vi "Three-PWM.vi"(8 "Error In":errorcluster, 11 "Dutycycle(%)":dbl[](array[numeric])) -> (0 "Error Out":errorcluster)   [LabVIEW 2019]
uses:
  <vilib>/Utility/error.llb/Error Cluster From Error Code.vi
  <vilib>/myRIO/Common/Instrument Driver Framework/myRIO v1.0/DIO/vis/myRIO v1.0 Write DIO.vi
  <vilib>/myRIO/Common/Instrument Driver Framework/myRIO v1.0/PWM/vis/myRIO v1.0 Write PWM.vi
  <vilib>/myRIO/Instrument Drivers/Onboard IO/PWM/PWM.lvlib
  <vilib>/myRIO/Instrument Drivers/Onboard IO/DIO/DIO.lvlib
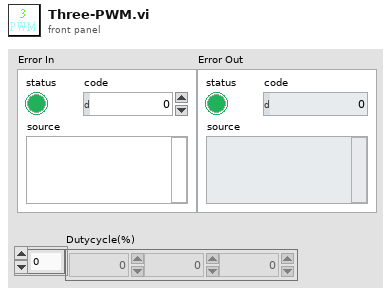
[diagram p1: front panel]
types:
  T1 = cluster{"馬達PWM腳位":tag, "馬達DIR腳位":tag[], "馬達Encoder角位":tag}[]
  T2 = cluster{"馬達PWM腳位":tag, "馬達DIR腳位":tag[], "馬達Encoder角位":tag}
  T3 = typedef "PWM.lvlib/PWM Reference.ctl" = cluster{"myRIO Reference":T4, "PWM Channels Enum":T8, "PWM Configuration":T9}
  T4 = typedef "myRIO Generic Hardware Reference.ctl" = cluster{"myRIO Model":T5, "myRIO Hardware Reference":T6}
  T5 = typedef "Hardware Version Enum.ctl" = enum16{"Unknown", "myRIO-1900", "myRIO-1950", "roboRIO", "NI ELVIS RIO CM", "ELVIS III"}
  T6 = typedef "myRIO v1.0 Reference.ctl" = cluster{"Generic FPGA Reference":T7, "Allow multiple opens":bool}
  T7 = typedef "Generic FPGA Reference.ctl" = refnum<k20>
  T8 = typedef "PWM Channels Enum.ctl" = enum16{"Not Connected", "C/PWM0", "C/PWM1", "A/PWM0", "A/PWM1", "A/PWM2", "A/PWM3", "A/PWM4", "A/PWM5", "A/PWM6", "A/PWM7", "A/PWM8", "A/PWM9", "A/PWM10", "A/PWM11", "A/PWM12", "A/PWM13", "A/PWM14", "A/PWM15", "A/PWM16", "A/PWM17", "A/PWM18", "A/PWM19", "B/PWM0", "B/PWM1", "B/PWM2", "B/PWM3", "B/PWM4", "B/PWM5", "B/PWM6", "B/PWM7", "B/PWM8", "B/PWM9", "B/PWM10", "B/PWM11", "B/PWM12", "B/PWM13", "B/PWM14", "B/PWM15", "B/PWM16", "B/PWM17", "B/PWM18", "B/PWM19", "PWM/PWM0", "PWM/PWM1", "PWM/PWM2", "PWM/PWM3", "PWM/PWM4", "PWM/PWM5", "PWM/PWM6", "PWM/PWM7", "PWM/PWM8", "PWM/PWM9"}
  T9 = typedef "PWM.lvlib/PWM Configuration.ctl" = cluster{"Frequency":dbl, "Duty Cycle":dbl}
  T10 = typedef "DIO.lvlib/DIO Reference.ctl" = cluster{"myRIO Reference":T4, "DIO Channels List":T11}
  T11 = typedef "DIO Channels List.ctl" = T12[]
  T12 = typedef "DIO Channels Enum.ctl" = enum16{"Not Connected", "C/DIO0", "C/DIO1", "C/DIO2", "C/DIO3", "C/DIO4", "C/DIO5", "C/DIO6", "C/DIO7", "A/DIO0", "A/DIO1", "A/DIO2", "A/DIO3", "A/DIO4", "A/DIO5", "A/DIO6", "A/DIO7", "A/DIO8", "A/DIO9", "A/DIO10", "A/DIO11", "A/DIO12", "A/DIO13", "A/DIO14", "A/DIO15", "A/DIO16", "A/DIO17", "A/DIO18", "A/DIO19", "B/DIO0", "B/DIO1", "B/DIO2", "B/DIO3", "B/DIO4", "B/DIO5", "B/DIO6", "B/DIO7", "B/DIO8", "B/DIO9", "B/DIO10", "B/DIO11", "B/DIO12", "B/DIO13", "B/DIO14", "B/DIO15", "B/DIO16", "B/DIO17", "B/DIO18", "B/DIO19", "LED0", "LED1", "LED2", "LED3", "Button0", "DIO/DIO0", "DIO/DIO1", "DIO/DIO2", "DIO/DIO3", "DIO/DIO4", "DIO/DIO5", "DIO/DIO6", "DIO/DIO7", "DIO/DIO8", "DIO/DIO9", "SPI/CS0", "SPI/CS1", "SPI/CS2", "SPI/CS3", "LED RADIO (Green)", "LED RADIO (Red)", "LED COMM (Green)", "LED COMM (Red)", "LED MODE (Green)", "LED MODE (Red)"}
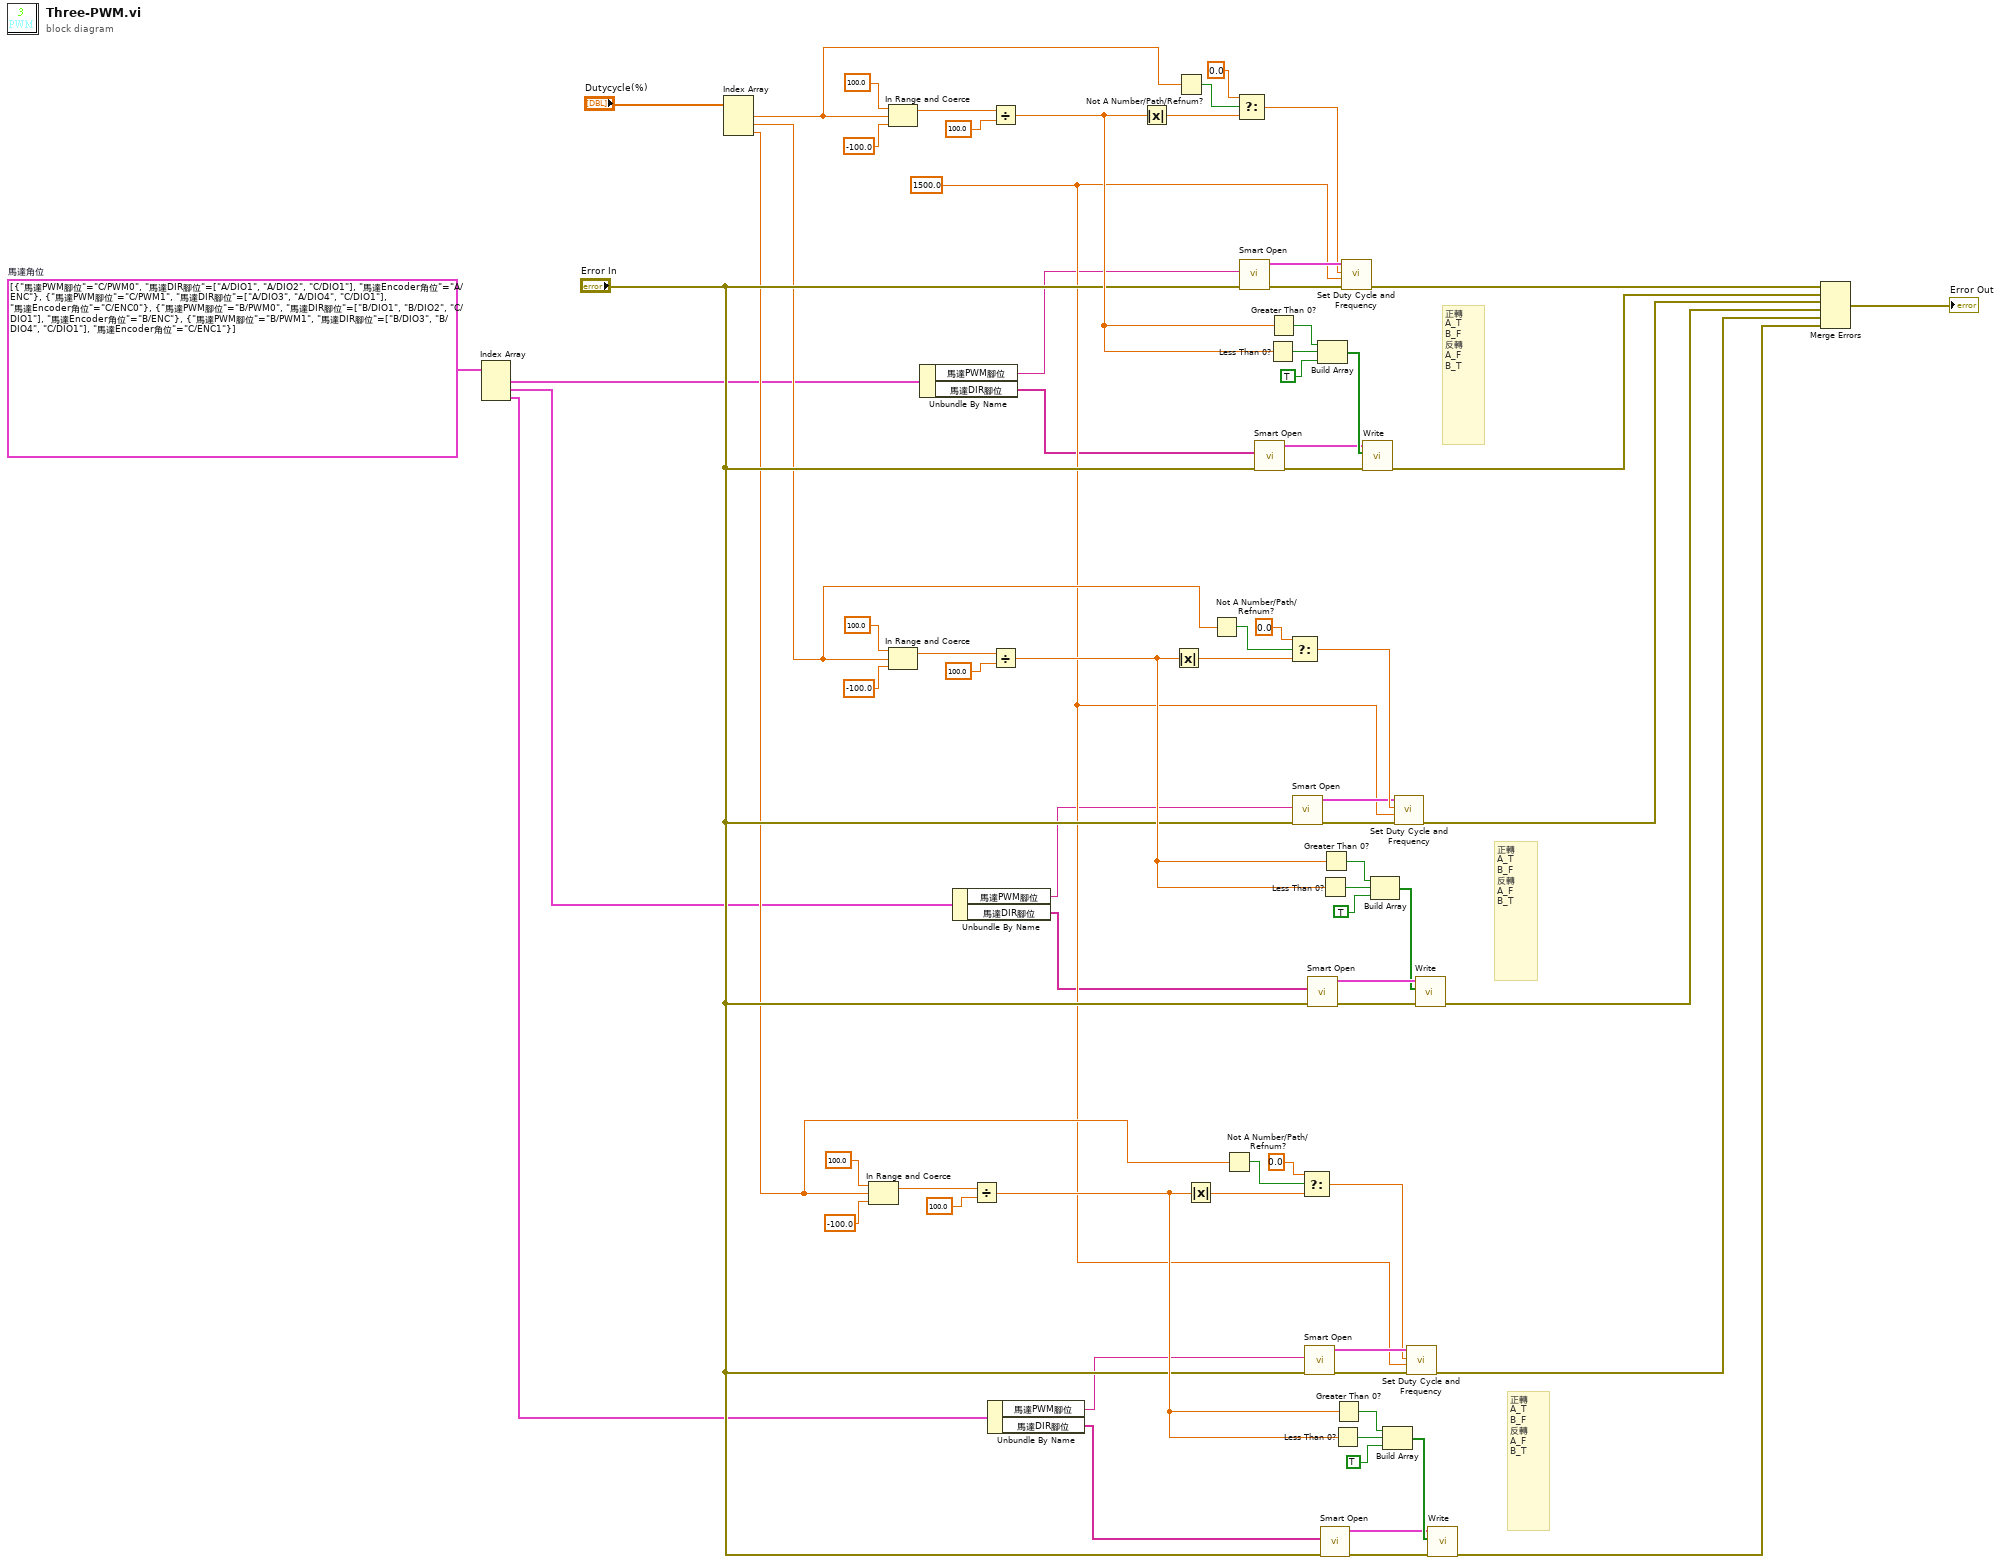
[diagram p0: block diagram]
diagram:
  w10 = T1 [{"馬達PWM腳位"="C/PWM0", "馬達DIR腳位"=["A/DIO1", "A/DIO2", "C/DIO1"], "馬達Encoder角位"="A/ENC"}, {"馬達PWM腳位"="C/PWM1", "馬達DIR腳位"=["A/DIO3", "A/DIO4", "C/DIO1"], "馬達Encoder角位"="C/ENC0"}, {"馬達PWM腳位"="B/PWM0", "馬達DIR腳位"=["B/DIO1", "B/DIO2", "C/DIO1"], "馬達Encoder角位"="B/ENC"}, {"馬達PWM腳位"="B/PWM1", "馬達DIR腳位"=["B/DIO3", "B/DIO4", "C/DIO1"], "馬達Encoder角位"="C/ENC1"}]  # 馬達角位
  w11 = 1500.0 ("Frequency [Hz]")
  # "正轉\nA_T\nB_F\n反轉\nA_F\nB_T"
  # "正轉\nA_T\nB_F\n反轉\nA_F\nB_T"
  # "正轉\nA_T\nB_F\n反轉\nA_F\nB_T"
  n1 = Index Array(array=w10) -> (element #1=w9:T2, element #2=w7:T2, element #3=w8:T2)  [unwired: 3 in]
  n2 = Index Array(array="Dutycycle(%)") -> (element #1=w14:dbl, element #2=w13:dbl, element #3=w12:dbl)  [unwired: 3 in]
  n3 = In Range and Coerce(upper limit=100.0, x=w12, lower limit=-100.0) -> (coerced(x)=w29:dbl)  [unwired: 1 out]
  n4 = In Range and Coerce(upper limit=100.0, x=w14, lower limit=-100.0) -> (coerced(x)=w63:dbl)  [unwired: 1 out]
  n5 = In Range and Coerce(upper limit=100.0, x=w13, lower limit=-100.0) -> (coerced(x)=w46:dbl)  [unwired: 1 out]
  n6 = Unbundle By Name(w9) -> ("馬達PWM腳位"=w5:tag, "馬達DIR腳位"=w6:tag[])
  n7 = Unbundle By Name(w7) -> ("馬達PWM腳位"=w3:tag, "馬達DIR腳位"=w4:tag[])
  n8 = Divide(x=w29, y=100.0) -> (x/y=w25:dbl)
  n9 = Unbundle By Name(w8) -> ("馬達PWM腳位"=w1:tag, "馬達DIR腳位"=w2:tag[])
  n10 = Divide(x=w63, y=100.0) -> (x/y=w59:dbl)
  n11 = Divide(x=w46, y=100.0) -> (x/y=w50:dbl)
  n12 = Absolute Value(x=w59) -> (abs(x)=w56:dbl)
  n13 = Absolute Value(x=w50) -> (abs(x)=w53:dbl)
  n14 = Not A Number/Path/Refnum?(number/path/refnum=w14) -> (NaN/Path/Refnum?=w58:bool)
  n15 = Absolute Value(x=w25) -> (abs(x)=w22:dbl)
  n16 = Not A Number/Path/Refnum?(number/path/refnum=w13) -> (NaN/Path/Refnum?=w51:bool)
  n17 = Not A Number/Path/Refnum?(number/path/refnum=w12) -> (NaN/Path/Refnum?=w24:bool)
  n18 = Select(t=0.0, s=w58, f=w56) -> (s? t:f=w55:dbl)
  n19 = call <vilib>:"Smart Open.vi"("error in (no error)"="Error In", "Channel Name"=w5) -> ("error out"=w73:errorcluster, "PWM Ref Out"=w74:T3)  [unwired: 8 in]
  n20 = call <vilib>:"Smart Open.vi"("error in (no error)"="Error In", "Channel Names"=w6) -> ("error out"=w70:errorcluster, "DIO Ref Out"=w71:T10)  [unwired: 8 in]
  n21 = Less Than 0?(x=w59) -> (x < 0?=w60:bool)
  n22 = Greater Than 0?(x=w59) -> (x > 0?=w61:bool)
  n23 = Select(t=0.0, s=w51, f=w53) -> (s? t:f=w54:dbl)
  n24 = call <vilib>:"Smart Open.vi"("error in (no error)"="Error In", "Channel Name"=w3) -> ("error out"=w39:errorcluster, "PWM Ref Out"=w38:T3)  [unwired: 8 in]
  n25 = Select(t=0.0, s=w24, f=w22) -> (s? t:f=w21:dbl)
  n26 = call <vilib>:"Smart Open.vi"("error in (no error)"="Error In", "Channel Name"=w1) -> ("error out"=w36:errorcluster, "PWM Ref Out"=w37:T3)  [unwired: 8 in]
  n27 = call <vilib>:"Smart Open.vi"("error in (no error)"="Error In", "Channel Names"=w4) -> ("error out"=w42:errorcluster, "DIO Ref Out"=w41:T10)  [unwired: 8 in]
  n28 = Build Array(w61, w60, TRUE) -> (w72:bool[])
  n29 = Less Than 0?(x=w50) -> (x < 0?=w49:bool)
  n30 = call <vilib>:"Smart Open.vi"("error in (no error)"="Error In", "Channel Names"=w2) -> ("error out"=w33:errorcluster, "DIO Ref Out"=w34:T10)  [unwired: 8 in]
  n31 = Greater Than 0?(x=w50) -> (x > 0?=w48:bool)
  n32 = Less Than 0?(x=w25) -> (x < 0?=w26:bool)
  n33 = Greater Than 0?(x=w25) -> (x > 0?=w27:bool)
  n34 = call <vilib>:"Set Duty Cycle and Frequency.vi"("error in (no error)"=w73, "Frequency [Hz]"=w11, "Duty Cycle"=w55, "PWM Ref In"=w74) -> ("error out"=w69:errorcluster)  [unwired: 5 in, 1 out]
  n35 = call <vilib>:"Write.vi"("error in (no error)"=w70, "Values"=w72, "DIO Ref In"=w71) -> ("error out"=w68:errorcluster)  [unwired: 6 in, 1 out]
  n36 = Build Array(w48, w49, TRUE) -> (w40:bool[])
  n37 = Build Array(w27, w26, TRUE) -> (w35:bool[])
  n38 = call <vilib>:"Set Duty Cycle and Frequency.vi"("error in (no error)"=w39, "Frequency [Hz]"=w11, "Duty Cycle"=w54, "PWM Ref In"=w38) -> ("error out"=w19:errorcluster)  [unwired: 5 in, 1 out]
  n39 = call <vilib>:"Set Duty Cycle and Frequency.vi"("error in (no error)"=w36, "Frequency [Hz]"=w11, "Duty Cycle"=w21, "PWM Ref In"=w37) -> ("error out"=w17:errorcluster)  [unwired: 5 in, 1 out]
  n40 = call <vilib>:"Write.vi"("error in (no error)"=w42, "Values"=w40, "DIO Ref In"=w41) -> ("error out"=w18:errorcluster)  [unwired: 6 in, 1 out]
  n41 = call <vilib>:"Write.vi"("error in (no error)"=w33, "Values"=w35, "DIO Ref In"=w34) -> ("error out"=w16:errorcluster)  [unwired: 6 in, 1 out]
  n42 = Merge Errors(w69, w68, w19, w18, w17, w16) -> (→"Error Out":errorcluster)
